vi "GetFieldFromProtobufIndex.vi"(1 "protobuf index":i32) -> (0 "oneof field name":string)   [LabVIEW 2021, in "NI DAQmx_server.lvlib" / "nidaqmx_grpc_GetChanAttributeStringRequest_attribute_enum.lvclass"]
uses:
  nidaqmx_grpc_GetChanAttributeStringRequest_attribute_enum.lvclass
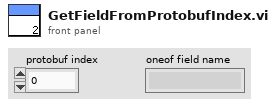
[diagram p1: front panel]
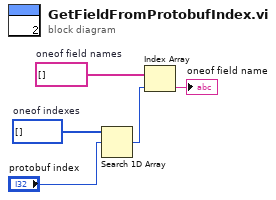
[diagram p0: block diagram]
diagram:
  w5 = string[] []  # oneof field names
  w4 = i32[] []  # oneof indexes
  n1 = Search 1D Array(1D array=w4, element="protobuf index") -> (index of element=w2:i32)  [unwired: 1 in]
  n2 = Index Array(array=w5, index=w2) -> (element=→"oneof field name":string)
